vi "Generate Trap Positiion Waveform.vi"(0 "Base trap positions":dbl[](array[numeric]), 1 "Data Period (s)":dbl, 2 "Input data":dbl[][](array[numeric]), 3 "Position calibration values":dbl[](array[numeric]), 4 "Trap Pos. Disp. Downsample (s)":dbl, 5 "Negate axis":bool[](array[boolean]), 8 "Time Stamp":timestamp) -> (6 "Output waveforms":waveform(dbl)[](array[waveform]), 7 "Output trap positions":cluster{"X":dbl[], "Y":dbl[]}[](array[cluster]))   [LabVIEW 2014]
uses:
  <vilib>/Analysis/baseanly.llb/Mean (DBL).vi
  <vilib>/Analysis/NI_AALBase.lvlib
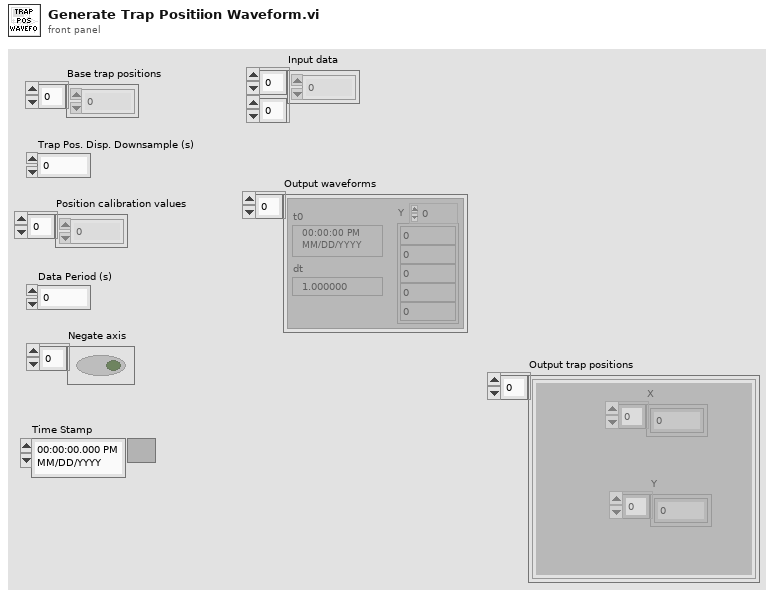
[diagram p1: front panel]
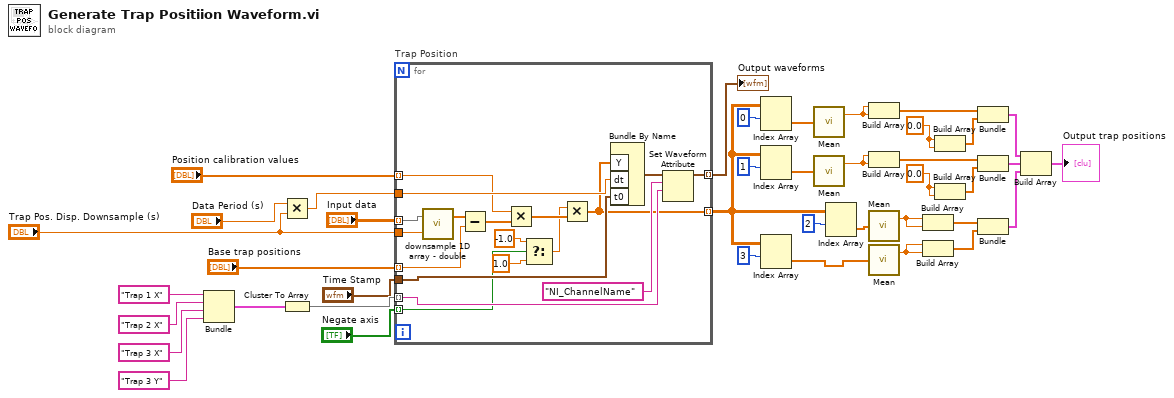
[diagram p0: block diagram]
diagram:
  w8 = 0.0
  w13 = 0.0
  n1 = Bundle("Trap 1 X", "Trap 2 X", "Trap 3 X", "Trap 3 Y") -> (w36:cluster{string, string, string, string})  [unwired: 1 out]
  n2 = Multiply(x="Data Period (s)", y="Trap Pos. Disp. Downsample (s)") -> (x*y=w40:dbl)
  n3 = Cluster To Array(cluster=w36) -> (array=w39:string[])
  n4 = for "Trap Position" {
    tunnel: "Input data" -> [w58] mode=indexing
    tunnel: "Trap Pos. Disp. Downsample (s)" -> [w57]
    tunnel: w40 -> [w55]
    tunnel: "Time Stamp" -> [w54]
    tunnel: w39 -> [w52] mode=indexing
    tunnel: [w51] -> w27 mode=indexing
    tunnel: "Base trap positions" -> [w49] mode=indexing
    tunnel: "Position calibration values" -> [w47] mode=indexing
    tunnel: "Negate axis" -> [w42] mode=indexing
    tunnel: [w41] -> w25 mode=indexing
    n5 = call "downsample 1D array - double.vi"("Ave N"=w57, "Array In"=w58) -> ("Array Out"=w56:dbl[])  [unwired: 1 out]
    n6 = Subtract(x=w56, y=w49) -> (x-y=w50:dbl[])
    n7 = Multiply(x=w47, y=w50) -> (x*y=w48:dbl[])
    n8 = Select(t=-1.0, s=w42, f=1.0) -> (s? t:f=w43:dbl)
    n9 = Multiply(x=w43, y=w48) -> (x*y=w41:dbl[])
    n10 = Bundle By Name("Y"=w41, "dt"=w55, "t0"=w54) -> (w53:waveform(dbl))  [unwired: 1 out]
    n11 = Set Waveform Attribute(5:w52, 6:"NI_ChannelName" ("name"), 7:w53) -> (3:w51:waveform(dbl))  [unwired: 1 in, 2 out]
  }
  "Output waveforms" <- w27
  n12 = Index Array(array=w25, index (row)=0) -> (element=w15:dbl[])  [unwired: 1 in]
  n13 = Index Array(array=w25, index (row)=1) -> (element=w16:dbl[])  [unwired: 1 in]
  n14 = Index Array(array=w25, index (row)=3) -> (element=w1:dbl[])  [unwired: 1 in]
  n15 = call-poly <vilib>:"Mean.vi"("X"=w15) -> ("mean"=w14:dbl)  [unwired: 1 out]
  n16 = call-poly <vilib>:"Mean.vi"("X"=w16) -> ("mean"=w12:dbl)  [unwired: 1 out]
  n17 = Index Array(array=w25, index (row)=2) -> (element=w17:dbl[])  [unwired: 1 in]
  n18 = Build Array(w14, w14) -> (w10:dbl[])
  n19 = Build Array(w12, w12) -> (w11:dbl[])
  n20 = call-poly <vilib>:"Mean.vi"("X"=w17) -> ("mean"=w6:dbl)  [unwired: 1 out]
  n21 = call-poly <vilib>:"Mean.vi"("X"=w1) -> ("mean"=w4:dbl)  [unwired: 1 out]
  n22 = Build Array(w6, w6) -> (w5:dbl[])
  n23 = Build Array(w4, w4) -> (w3:dbl[])
  n24 = Build Array(w13, w13) -> (w9:dbl[])
  n25 = Build Array(w8, w8) -> (w7:dbl[])
  n26 = Bundle(w10, w9) -> (w24:cluster{dbl[], dbl[]})  [unwired: 1 in]
  n27 = Bundle(w11, w7) -> (w23:cluster{dbl[], dbl[]})  [unwired: 1 in]
  n28 = Bundle(w5, w3) -> (w22:cluster{dbl[], dbl[]})  [unwired: 1 in]
  n29 = Build Array(w24, w23, w22) -> (→"Output trap positions":cluster{dbl[], dbl[]}[])
